vi "Read Power.vi"(0 "SG Path Power Meter Accessor in":refnum<class "SG Path Accessor.lvclass">, 5 "Cal point in":T1, 11 "error in (no error)":errorcluster) -> (4 "SG Path Power Meter Accessor out":refnum<class "SG Path Accessor.lvclass">, 6 "Power (dBm)":dbl, 15 "error out":errorcluster)   [LabVIEW 2023, in "NI-568x RF Power Meter.lvlib" / "SG Path Accessor.lvclass"]
uses:
  SG Path Accessor.lvclass
  Public/Base Classes/Scalar/Scalar Path/Type Definitions/Cal Point.ctl
  Power Meter/Power Meter.lvclass
  Power Meter/Power Meter.lvclass/Power Meter.ctl
  Power Meter/Properties/Read Resource Name.vi
  <instrlib>/ni568x/ni568x.llb/ni568x Read.vi
  Instruments/Power Meter/Power Meter Factory/Power Meter Factory.lvclass
  Public/Base Classes/Scalar/Scalar Path/Scalar Path.lvclass
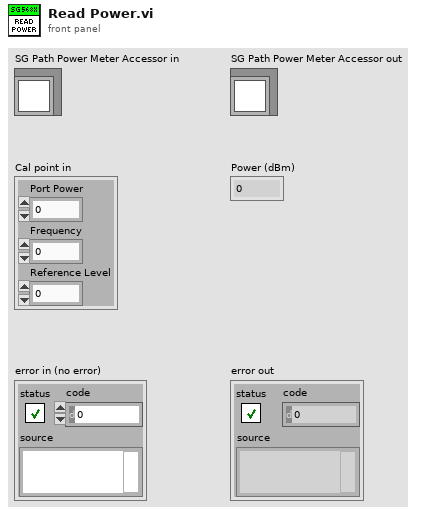
[diagram p1: front panel]
types:
  T1 = typedef "RFFixtureCharact.Public.lvlib/Scalar Path.lvclass/Cal Point.ctl" = cluster{"Port Power":dbl, "Frequency":dbl, "Reference Level":dbl}
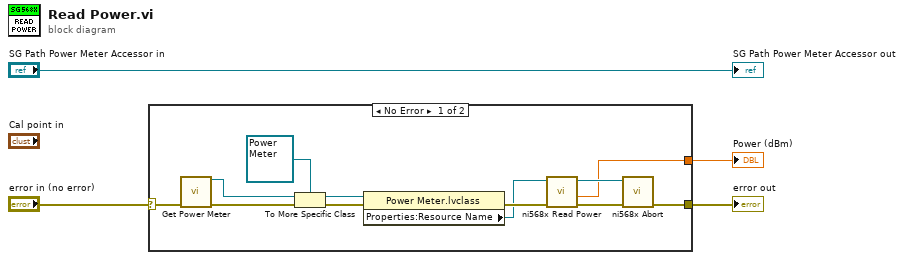
[diagram p0: block diagram]
diagram:
  n1 = case shown="No Error" "error in (no error)" {
    selector: "error in (no error)" -> [w16 w17]
    tunnel: [w5 w17] -> w4
    tunnel: [w6 _] -> w2
    frame No Error {
      n2 = call "Get Power Meter.vi"("error in (no error)"=w16) -> ("Power Meter Base out"=w8:refnum<class "Power Meter Base.lvclass">, "error out"=w7:errorcluster)  [unwired: 13 in]
      n3 = To More Specific Class(target class=refnum<class "Power Meter.lvclass"> refnum ("PM NI568X in"), reference=w8, error in=w7) -> (specific class reference=w11:refnum<class "Power Meter.lvclass">, error out=w13:errorcluster)
      n4 = property class="Power Meter.lvclass"(reference=w11, error in=w13) -> (error out=w12:errorcluster, "Properties:Resource Name"=w10:refnum<k15>)  [unwired: 1 out]
      n5 = call-poly <instrlib>:"ni568x Read Power.vi"("error in"=w12, "instrument handle"=w10) -> ("error out"=w15:errorcluster, "power"=w6:dbl, "instrument handle out"=w14:refnum<k15>)  [unwired: 7 in]
      n6 = call <instrlib>:"ni568x Abort.vi"("error in"=w15, "instrument handle"=w14) -> ("error out"=w5:errorcluster)  [unwired: 8 in, 1 out]
    }
    frame Error {
    }
  }
  "error out" <- w4
  "Power (dBm)" <- w2
  "SG Path Power Meter Accessor out" <- "SG Path Power Meter Accessor in"
